vi "NXT Camera Test2.vi"() -> ()   [LabVIEW 2016]
uses:
  <vilib>/NXT/Block Support/NXT_InputPort.ctl
  <vilib>/NXT/Block Support/NXT_OutputPort.ctl
  <vilib>/NXT/Dual Mode Library/prims/inRangeAndCoerce/inRangeAndCoerce_int8.vi
  <vilib>/NXT/NXTIO Xnodes/NXTIONodeSubVIs/NXTMoveMotors.vi
  <vilib>/NXT/NXTIO Xnodes/NXTIONodeSubVIs/NXTStopMotors.vi
  <vilib>/NXT/Subs/LVHSConnector.ctl
  <vilib>/NXT/NXTIO Xnodes/AddressXNode/NXTIOAddress.xnode
  <vilib>/NXT/NXTIO Xnodes/NXTIOXNode/NXTIO.xnode
  <vilib>/NXT/LegoClasses/BrickReference/BrickReference.lvclass
panel:
  in  "stop":bool
  out "Power":bool
  out "X Upper Left":u8
  out "X Lower Right":u8
  out "Y Lower Right":u8
  out "Y Upper Left":u8
  out "Count":u8
  out "Color":u8
  in  "Cluster":T1 {"Tracking Mode" items=["Disable Tracking", "Get First Object", "Get n th Object", "Enable Tracking", "Sort Objects  by size", "Sort Objects  by Colors", "Illumination on ", "Illumination Off", "Write Colormap", "Read Colormap", "Line tracking mode", "Object Tracking mode"]}
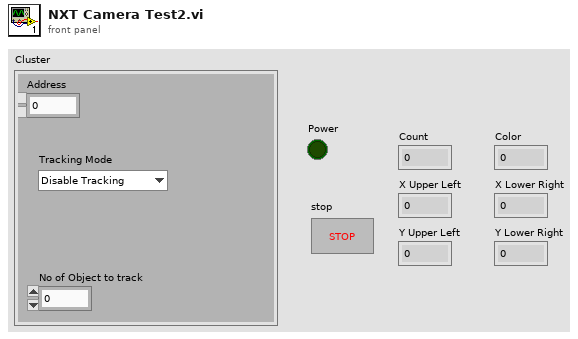
[diagram p1: front panel]
types:
  T1 = cluster{"Address":dbl, "No of Object to track":dbl, "Tracking Mode":u8}
  T2 = cluster{"Tracking Mode":u8, "Object Number to Track":u8, "Address":u8}
  T3 = typedef "NXT_InputPort.ctl" = u32
  T4 = typedef "LVHSConnector.ctl" = refnum<class "BrickReference.lvclass">
  T5 = cluster{"Total Tracked Objects":u8, "Color":u8, "X Upper Left":u8, "Y Upper Left":u8, "X Lower Right":u8, "Y Lower Right":u8, "Status (boolean)":bool}
  T6 = typedef "NXT_OutputPort.ctl" = u8
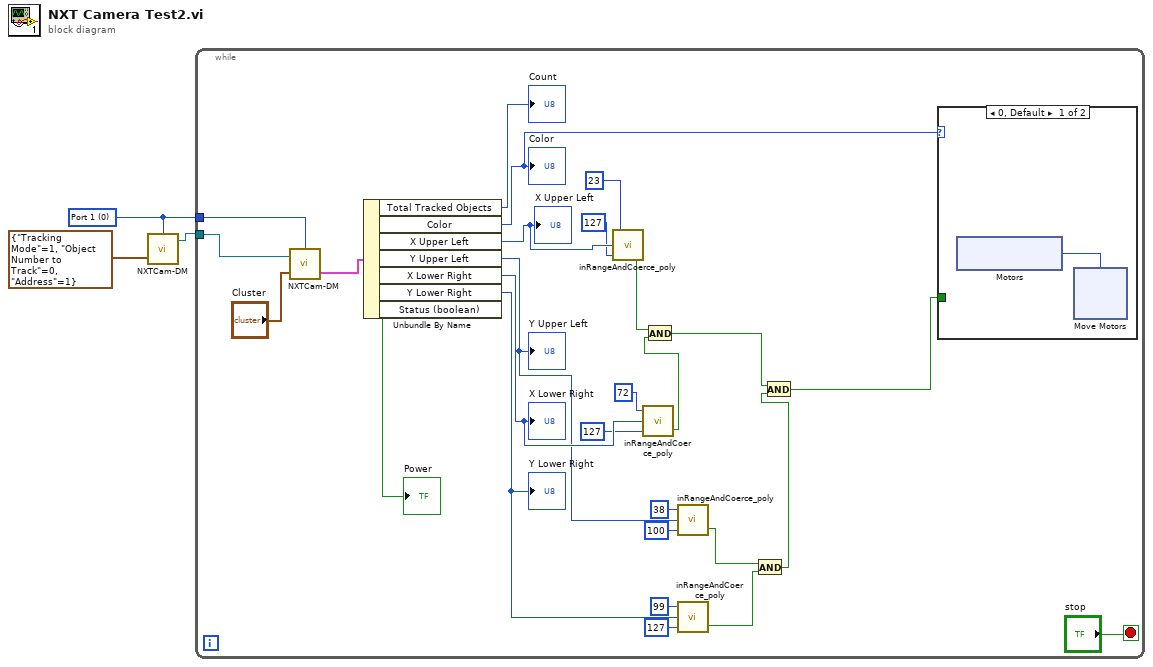
[diagram p0: block diagram]
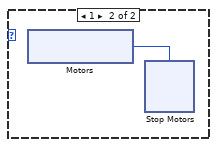
[diagram p2: hidden frame]
diagram:
  w1 = T3 0 items=["Port 1", "Port 2", "Port 3", "Port 4"] ("Input Port")
  n1 = call "NXTCam-DM.vi"("Input of NXTCam"=T2 {"Tracking Mode"=1, "Object Number to Track"=0, "Address"=1}, "Input Port"=w1) -> ("NXT dup"=w3:T4)  [unwired: 1 in, 1 out]
  n2 = while {
    tunnel: w1 -> [w27]
    tunnel: w3 -> [w25]
    stop <- "stop" stop-if-true
    n3 = call "NXTCam-DM.vi"("Input of NXTCam"="Cluster", "NXT"=w25, "Input Port"=w27) -> ("Output of NXTCam"=w26:T5)  [unwired: 1 out]
    n4 = Unbundle By Name(w26) -> ("Total Tracked Objects"=→"Count":u8, "Color"=w23:u8, "X Upper Left"=w22:u8, "Y Upper Left"=w14:u8, "X Lower Right"=w19:u8, "Y Lower Right"=w11:u8, "Status (boolean)"=→"Power":bool)
    "X Upper Left" <- w22
    "X Lower Right" <- w19
    "Y Lower Right" <- w11
    "Y Upper Left" <- w14
    "Color" <- w23
    n5 = call-poly <vilib>:"inRangeAndCoerce_poly.vi"("lower limit"=i8 127, "x"=w22, "upper limit"=i8 23) -> ("In Range?"=w15:bool)  [unwired: 1 out]
    n6 = call-poly <vilib>:"inRangeAndCoerce_poly.vi"("lower limit"=i8 127, "x"=w19, "upper limit"=i8 72) -> ("In Range?"=w16:bool)  [unwired: 1 out]
    n7 = And(x=w15, y=w16) -> (x .and. y?=w5:bool)
    n8 = call-poly <vilib>:"inRangeAndCoerce_poly.vi"("lower limit"=i8 100, "x"=w14, "upper limit"=i8 38) -> ("In Range?"=w8:bool)  [unwired: 1 out]
    n9 = call-poly <vilib>:"inRangeAndCoerce_poly.vi"("lower limit"=i8 127, "x"=w11, "upper limit"=i8 99) -> ("In Range?"=w7:bool)  [unwired: 1 out]
    n10 = And(x=w8, y=w7) -> (x .and. y?=w6:bool)
    n11 = And(x=w5, y=w6) -> (x .and. y?=w4:bool)
    n12 = case shown="0, Default" w23 {
      tunnel: w4 -> [_ _]
      frame 0, Default {
        n13 = xnode "Motors"() -> ("Motor"=w31:T6)
        n14 = xnode "Move Motors"("Motors"=w31) -> ()  [unwired: 2 in, 1 out]
      }
      frame 1 {
        n15 = xnode "Motors"() -> ("Motor"=w40:T6)
        n16 = xnode "Stop Motors"("Motors"=w40) -> ()  [unwired: 1 in, 1 out]
      }
    }
  }
